vi "sonar test.vi"() -> ()   [LabVIEW 2011]
panel:
  out "Numeric Indicator":dbl
  in  "stop":bool
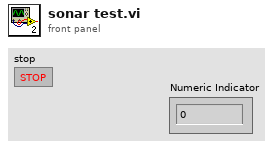
[diagram p1: front panel]
types:
  T1 = typedef "WPI_AnalogChannelDevRef.ctl" = cluster{"DevStatus":errorcluster, "Analog Module":T2, "Analog Channel":T3}
  T2 = typedef "FPGA_TypedefAnalogModule.ctl" = enum16{"Analog Module 1", "Analog Module 2"}
  T3 = typedef "FPGA_AIChannel.ctl" = enum8{"AI 1", "AI 2", "AI 3", "AI 4", "AI 5", "AI 6", "AI 7", "AI 8", "Invalid"}
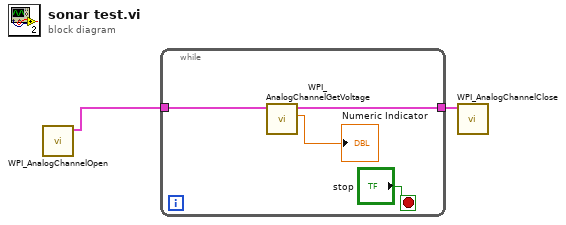
[diagram p0: block diagram]
diagram:
  n1 = call <vilib>:"WPI_AnalogChannelOpen.vi"() -> ("AIDeviceRef"=w2:T1)  [unwired: 10 in, 1 out]
  n2 = while {
    tunnel: w2 -> [w5]
    tunnel: [w4] -> w1
    stop <- "stop" stop-if-true
    n3 = call <vilib>:"WPI_AnalogChannelGetVoltage.vi"("AIDeviceRef"=w5) -> ("Voltage"=→"Numeric Indicator":dbl, "AIDeviceRef"=w4:T1)  [unwired: 8 in, 1 out]
  }
  n4 = call <vilib>:"WPI_AnalogChannelClose.vi"("AIDeviceRef"=w1) -> ()  [unwired: 10 in, 1 out]
